vi "Select File.vi"(8 "error in (no error)":errorcluster, 9 "File Path Control":path, 11 "Setup File in":refnum<class "Setup File.lvclass">) -> (0 "error out":errorcluster, 3 "Setup File out":refnum<class "Setup File.lvclass">)   [LabVIEW 2018, in "Setup File.lvclass"]
doc: "Este VI recebe o caminho de um arquivo e salva na classe, em formato string, o nome e caminho desse arquivo."
uses:
  Setup File.lvclass
  Setup File.lvclass/Setup File.ctl
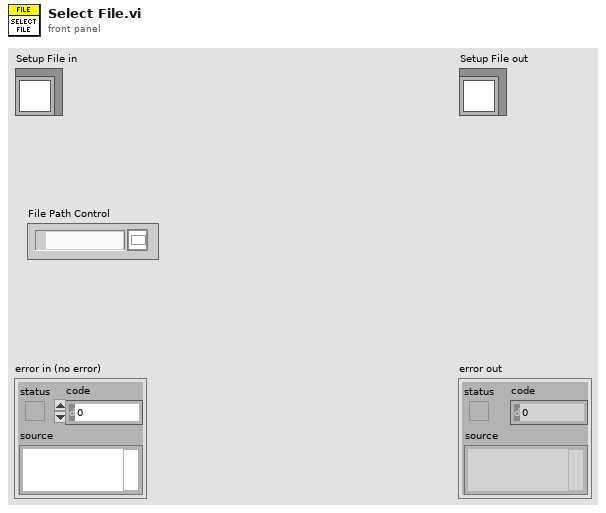
[diagram p1: front panel]
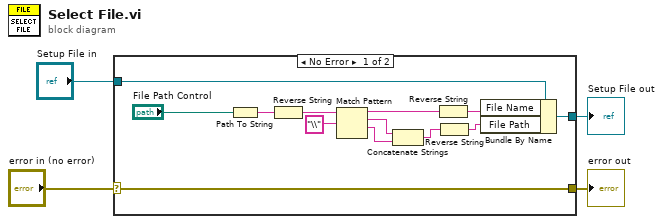
[diagram p0: block diagram]
diagram:
  n1 = case shown="No Error" "error in (no error)" {
    selector: "error in (no error)" -> [w17 w19]
    tunnel: [w17 w19] -> w3
    tunnel: [w14 w18] -> w1
    tunnel: "Setup File in" -> [w15 w18]
    frame No Error {
      n2 = Path To String(path="File Path Control") -> (string=w13:string)
      n3 = Reverse String(1:w13) -> (0:w12:string)
      n4 = Match Pattern(string=w12, regular expression="\\") -> (before substring=w9:string, match substring=w5:string, after substring=w6:string)  [unwired: 1 in, 1 out]
      n5 = Concatenate Strings(w5, w6) -> (w8:string)
      n6 = Reverse String(1:w9) -> (0:w11:string)
      n7 = Reverse String(1:w8) -> (0:w10:string)
      n8 = Bundle By Name(cluster=w15, "File Name"=w11, "File Path"=w10) -> (w14:refnum<class "Setup File.lvclass">)
    }
    frame Error {
    }
  }
  "error out" <- w3
  "Setup File out" <- w1
